vi "VGI Read Board Info.vi"(8 "error in (no error)":errorcluster, 11 "DevIndex":i32) -> (0 "error out":errorcluster, 2 "function return":i32, 3 "pInfo":T1)   [LabVIEW 2012, in "ControlGPIO.lvlib"]
doc: "int WINAPI VGI_ReadBoardInfo(int DevIndex,PVGI_BOARD_INFO pInfo);"
uses:
  ControlGPIO.lvlib
  Ginkgo_Driver.dll
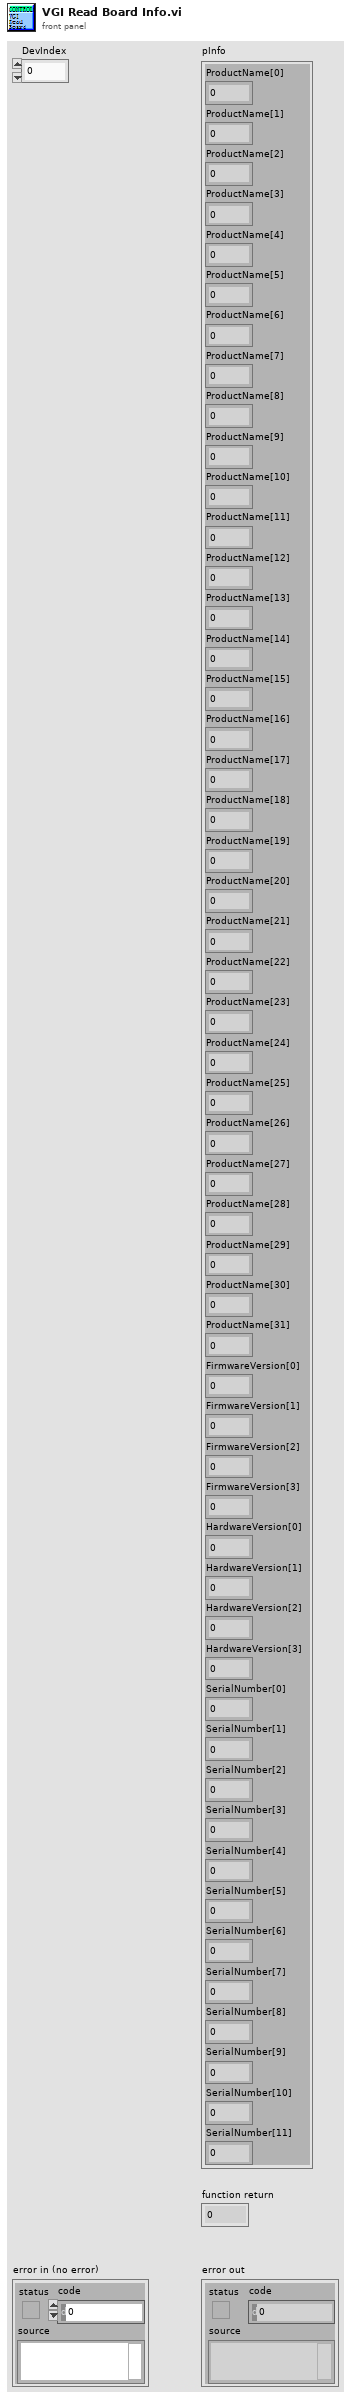
[diagram p1: front panel]
types:
  T1 = cluster{"ProductName[0]":u8, "ProductName[1]":u8, "ProductName[2]":u8, "ProductName[3]":u8, "ProductName[4]":u8, "ProductName[5]":u8, "ProductName[6]":u8, "ProductName[7]":u8, "ProductName[8]":u8, "ProductName[9]":u8, "ProductName[10]":u8, "ProductName[11]":u8, "ProductName[12]":u8, "ProductName[13]":u8, "ProductName[14]":u8, "ProductName[15]":u8, "ProductName[16]":u8, "ProductName[17]":u8, "ProductName[18]":u8, "ProductName[19]":u8, "ProductName[20]":u8, "ProductName[21]":u8, "ProductName[22]":u8, "ProductName[23]":u8, "ProductName[24]":u8, "ProductName[25]":u8, "ProductName[26]":u8, "ProductName[27]":u8, "ProductName[28]":u8, "ProductName[29]":u8, "ProductName[30]":u8, "ProductName[31]":u8, "FirmwareVersion[0]":u8, "FirmwareVersion[1]":u8, "FirmwareVersion[2]":u8, "FirmwareVersion[3]":u8, "HardwareVersion[0]":u8, "HardwareVersion[1]":u8, "HardwareVersion[2]":u8, "HardwareVersion[3]":u8, "SerialNumber[0]":u8, "SerialNumber[1]":u8, "SerialNumber[2]":u8, "SerialNumber[3]":u8, "SerialNumber[4]":u8, "SerialNumber[5]":u8, "SerialNumber[6]":u8, "SerialNumber[7]":u8, "SerialNumber[8]":u8, "SerialNumber[9]":u8, "SerialNumber[10]":u8, "SerialNumber[11]":u8}
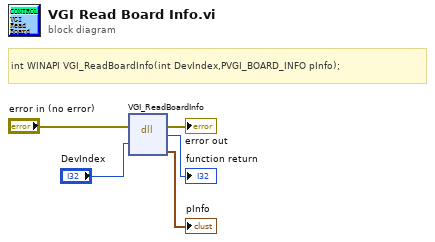
[diagram p0: block diagram]
diagram:
  # "int WINAPI VGI_ReadBoardInfo(int DevIndex,PVGI_BOARD_INFO pInfo);"
  n1 = dll-call lib="E:/Project/vt_ginkgo/truck/Ginkgo Driver/vs2010/Ginkgo_USB-I2C_API_v2.0.3.0/lib/labview_64bit/ControlGPIO/Ginkgo_Driver.*" fn="VGI_ReadBoardInfo"(error in="error in (no error)", "DevIndex"="DevIndex") -> (error out=→"error out":errorcluster, →"function return":i32, "pInfo"=→"pInfo":T1)  [unwired: 4 in, 1 out]
